vi "FT_Reset_Device.vi"(8 "error in":errorcluster, 11 "Handle":u32) -> (0 "error out":errorcluster, 3 "Handle out":u32)   [LabVIEW 2016]
uses:
  FTD2XX.dll
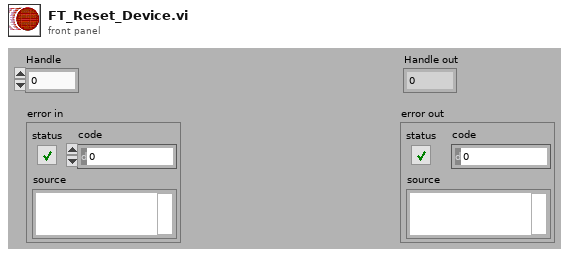
[diagram p1: front panel]
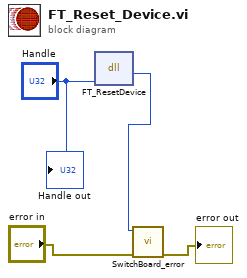
[diagram p0: block diagram]
diagram:
  n1 = dll-call lib="FTD2XX.dll" fn="FT_ResetDevice"("Handle"="Handle") -> ("FT_Status"=w1:u32)  [unwired: 4 in, 2 out]
  n2 = call <instrlib>:"SwitchBoard_error.vi"("error constant"="error in", "Code"=w1) -> ("error IO"=→"error out":errorcluster)  [unwired: 9 in]
  "Handle out" <- "Handle"
